vi "create T list.vi"(2 "mod set list":bool, 7 "exp exec in":T2={"data file"={"autosave"=FALSE, "File refnum"=refnum, "data file path"=path ""}, "T log file"={"File refnum"=refnum, "T log file path"=path "", "exists"=FALSE}, "exp seq"={"wave params"={"Num of avg"=0, "Num points"=1000, "Meas rate (Hz)"=100000.0}, "Setpoints"=[], "#"=-1, "index"=-1, "elapsed time (s)"=0.0, "set time (s)"=0.0, "min settle (s)"=30.0, " Exec Status"=enum."Settling"}, "error"={"status"=FALSE, "code"=0, "source"=""}}, 12 "wave params":T1={"Num of avg"=100, "Num points"=1000, "Meas rate (Hz)"=100000.0} caption="waveform parameters") -> (8 "exp exec out":T2={"data file"={"autosave"=FALSE, "File refnum"=refnum, "data file path"=path ""}, "T log file"={"File refnum"=refnum, "T log file path"=path "", "exists"=FALSE}, "exp seq"={"wave params"={"Num of avg"=0, "Num points"=1000, "Meas rate (Hz)"=100000.0}, "Setpoints"=[], "#"=-1, "index"=-1, "elapsed time (s)"=0.0, "set time (s)"=0.0, "min settle (s)"=30.0, " Exec Status"=enum."Settling"}, "error"={"status"=FALSE, "code"=0, "source"=""}}, 14 "Setpoints":dbl[](array[numeric]) caption="Setpoint List", 15 "N Sets":i32 caption="Num of Setpoints")   [LabVIEW 2019]
doc: "This is a Bug C(T) subVI.\n\nIt is a container for the setpoint list generation popup.\n\nPaul K Dixon\nP3600\nCSUSB Physics"
uses:
  typedefs/PID exec cluster.ctl
  typedefs/data file info.ctl
  typedefs/bug temp file info.ctl
  typedefs/exp seq cluster.ctl
  typedefs/wvfm acq params.ctl
  typedefs/bug meas status.ctl
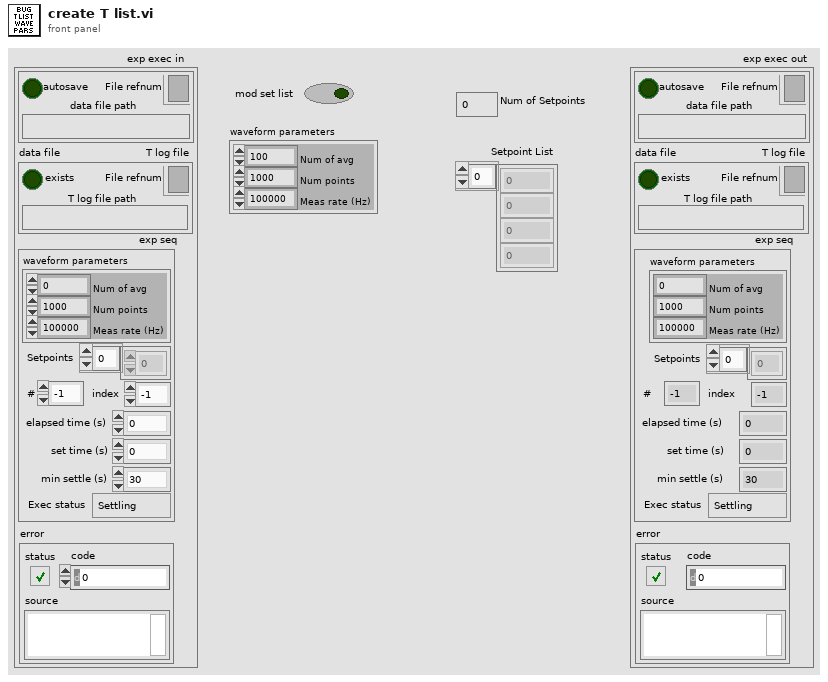
[diagram p1: front panel]
types:
  T1 = typedef "wvfm acq params.ctl" = cluster{"Num of avg":i32, "Num points":i32, "Meas rate (Hz)":dbl}
  T2 = typedef "PID exec cluster.ctl" = cluster{"data file":T3, "T log file":T4, "exp seq":T5, "error":errorcluster}
  T3 = typedef "data file info.ctl" = cluster{"autosave":bool, "File refnum":refnum<file>, "data file path":path}
  T4 = typedef "bug temp file info.ctl" = cluster{"File refnum":refnum<file>, "T log file path":path, "exists":bool}
  T5 = typedef "exp seq cluster.ctl" = cluster{"wave params":T1, "Setpoints":dbl[], "#":i32, "index":i32, "elapsed time (s)":dbl, "set time (s)":dbl, "min settle (s)":dbl, " Exec Status":T6}
  T6 = typedef "bug meas status.ctl" = enum32{"Settling", "Measuring", "Holding", "Exit"}
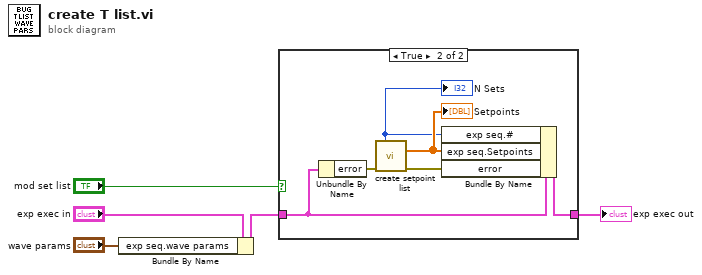
[diagram p0: block diagram]
diagram:
  n1 = Bundle By Name(cluster="exp exec in", "exp seq.wave params"="wave params") -> (w2:T2)
  n2 = case shown="True" "mod set list" {
    tunnel: w2 -> [w6 w12]
    tunnel: [w6 w10] -> w5
    frame False {
    }
    frame True {
      n3 = Unbundle By Name(w12) -> ("error"=w11:errorcluster)
      n4 = call "create setpoint list.vi"("error in (no error)"=w11) -> ("N points"=w7:i32, "Setpoint array"=w8:dbl[], "error out"=w9:errorcluster)  [unwired: 12 in]
      "Setpoints" <- w8
      "N Sets" <- w7
      n5 = Bundle By Name(cluster=w12, "exp seq.#"=w7, "exp seq.Setpoints"=w8, "error"=w9) -> (w10:T2)
    }
  }
  "exp exec out" <- w5
